vi "Check Color Range Change.vi"(9 "Color Range in":T1={"Hue"={46, 0.0}, "Sat"={0, 0.0}, "Val"={0, 0.0}}, 11 "Name":string="Port Color Range") -> (1 "Color Range out":T1={"Hue"={46, 0.0}, "Sat"={0, 0.0}, "Val"={0, 0.0}}, 3 "Changed":bool)   [LabVIEW 2025]
uses:
  <vilib>/Rock Robotics/Network Tables/NT Read Integer Array.vi
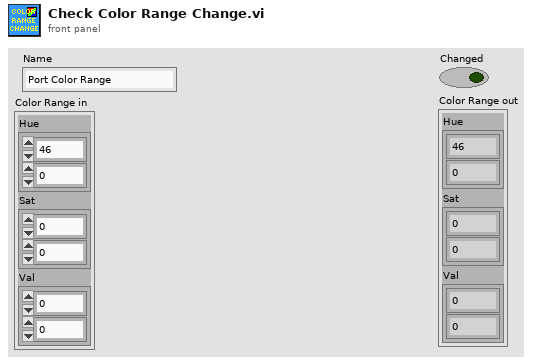
[diagram p1: front panel]
types:
  T1 = cluster{"Hue":cluster{i64, dbl}, "Sat":cluster{i64, dbl}, "Val":cluster{i64, dbl}}
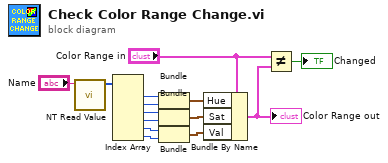
[diagram p0: block diagram]
diagram:
  n1 = call-poly <vilib>:"NT Read Value.vi"("name"="Name") -> ("value"=w11:i64[])  [unwired: 8 in, 2 out]
  n2 = Index Array(array=w11) -> (element #1=w10:i64, element #2=w9:i64, element #3=w8:i64, element #4=w7:i64, element #5=w6:i64, element #6=w5:i64)  [unwired: 6 in]
  n3 = Bundle("Numeric"=w10, "Numeric"=w9) -> (w4:cluster{"Numeric":i64, "Numeric":i64})  [unwired: 1 in]
  n4 = Bundle("Numeric"=w8, "Numeric"=w7) -> (w3:cluster{"Numeric":i64, "Numeric":i64})  [unwired: 1 in]
  n5 = Bundle("Numeric"=w6, "Numeric"=w5) -> (w2:cluster{"Numeric":i64, "Numeric":i64})  [unwired: 1 in]
  n6 = Bundle By Name(cluster="Color Range in", "Hue"=w4, "Sat"=w3, "Val"=w2) -> (w1:T1)
  "Color Range out" <- w1
  n7 = Not Equal?(x="Color Range in", y=w1) -> (x != y?=→"Changed":bool)
